vi "Drive Core.vi"(0 "A Encoder BL":string="My Motor RefNum", 1 "Rotational Motor FR":string="My Motor RefNum", 2 "Rotational Motor FL":string="My Motor RefNum", 3 "Rotational Motor BR":string="My Motor RefNum", 4 "Rotational Motor BL":string="My Motor RefNum", 5 "Drive Motor FR":string="My Motor RefNum", 6 "A Encoder BR":string="My Motor RefNum", 7 "Drive Motor FL":string="My Motor RefNum", 8 "A Encoder FL":string="My Motor RefNum", 9 "Drive Motor BR":string="My Motor RefNum", 10 "A Encoder FR":string="My Motor RefNum", 11 "Drive Motor BL":string="My Motor RefNum") -> ()   [LabVIEW 2014]
uses:
  Global Variables.vi
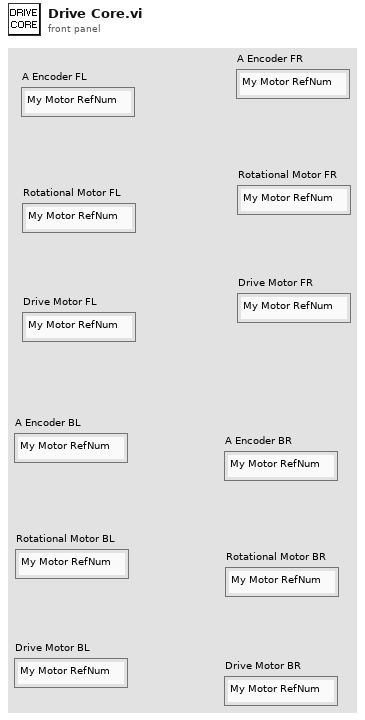
[diagram p1: front panel]
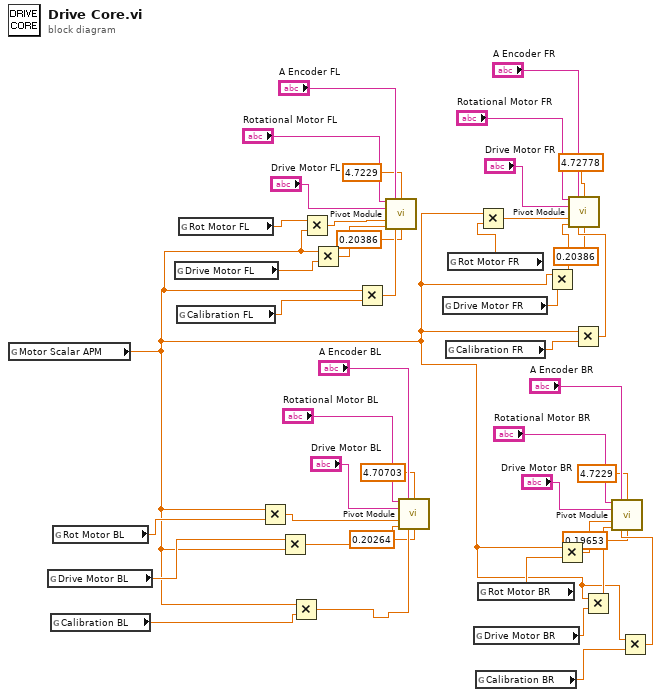
[diagram p0: block diagram]
diagram:
  n1 = global read "Global Variables.vi" "Motor Scalar APM"() -> (w10:dbl)
  n2 = global read "Global Variables.vi" "Drive Motor BL"() -> (w25:dbl)
  n3 = global read "Global Variables.vi" "Calibration BL"() -> (w27:dbl)
  n4 = global read "Global Variables.vi" "Rot Motor BL"() -> (w22:dbl)
  n5 = global read "Global Variables.vi" "Drive Motor FL"() -> (w31:dbl)
  n6 = global read "Global Variables.vi" "Calibration FL"() -> (w33:dbl)
  n7 = global read "Global Variables.vi" "Rot Motor FL"() -> (w29:dbl)
  n8 = Multiply(x=w10, y=w22) -> (x*y=w23:dbl)
  n9 = Multiply(x=w25, y=w10) -> (x*y=w24:dbl)
  n10 = Multiply(x=w10, y=w27) -> (x*y=w26:dbl)
  n11 = Multiply(x=w29, y=w10) -> (x*y=w28:dbl)
  n12 = Multiply(x=w10, y=w31) -> (x*y=w30:dbl)
  n13 = Multiply(x=w10, y=w33) -> (x*y=w32:dbl)
  n14 = call "Pivot Module.vi"("Rotational Motor Refnum"="Rotational Motor FL", "Encoder Refnum"="A Encoder FL", "Top Voltage"=4.7229, "Drive Motor Refnum"="Drive Motor FL", "Motor Angle"=w28, "Motor Speed"=w30, "Calibration Angle"=w32, "Bottom Voltage"=0.20386) -> ()  [unwired: 8 in]
  n15 = call "Pivot Module.vi"("Rotational Motor Refnum"="Rotational Motor BL", "Encoder Refnum"="A Encoder BL", "Top Voltage"=4.70703, "Drive Motor Refnum"="Drive Motor BL", "Motor Angle"=w23, "Motor Speed"=w24, "Calibration Angle"=w26, "Bottom Voltage"=0.20264) -> ()  [unwired: 8 in]
  n16 = global read "Global Variables.vi" "Drive Motor FR"() -> (w19:dbl)
  n17 = global read "Global Variables.vi" "Calibration FR"() -> (w17:dbl)
  n18 = global read "Global Variables.vi" "Rot Motor FR"() -> (w21:dbl)
  n19 = global read "Global Variables.vi" "Drive Motor BR"() -> (w13:dbl)
  n20 = global read "Global Variables.vi" "Calibration BR"() -> (w11:dbl)
  n21 = Multiply(x=w10, y=w21) -> (x*y=w20:dbl)
  n22 = global read "Global Variables.vi" "Rot Motor BR"() -> (w15:dbl)
  n23 = Multiply(x=w10, y=w19) -> (x*y=w18:dbl)
  n24 = Multiply(x=w10, y=w15) -> (x*y=w14:dbl)
  n25 = Multiply(x=w10, y=w17) -> (x*y=w16:dbl)
  n26 = call "Pivot Module.vi"("Rotational Motor Refnum"="Rotational Motor FR", "Encoder Refnum"="A Encoder FR", "Top Voltage"=4.72778, "Drive Motor Refnum"="Drive Motor FR", "Motor Angle"=w20, "Motor Speed"=w18, "Calibration Angle"=w16, "Bottom Voltage"=0.20386) -> ()  [unwired: 8 in]
  n27 = Multiply(x=w10, y=w13) -> (x*y=w12:dbl)
  n28 = Multiply(x=w10, y=w11) -> (x*y=w9:dbl)
  n29 = call "Pivot Module.vi"("Rotational Motor Refnum"="Rotational Motor BR", "Encoder Refnum"="A Encoder BR", "Top Voltage"=4.7229, "Drive Motor Refnum"="Drive Motor BR", "Motor Angle"=w14, "Motor Speed"=w12, "Calibration Angle"=w9, "Bottom Voltage"=0.19653) -> ()  [unwired: 8 in]
